vi "Read & Write Visa.vi"(8 "error in (no error)":errorcluster, 10 "Message":string, 11 "VISA Refnum in":refnum<visa-resource-name>) -> (0 "error out":errorcluster, 2 "read buffer":string, 3 "VISA Refnum out":refnum<visa-resource-name>)   [LabVIEW 2022 SP3]
uses:
  42f06f77-e9dd-42f2-8331-d96ccd674586.vi
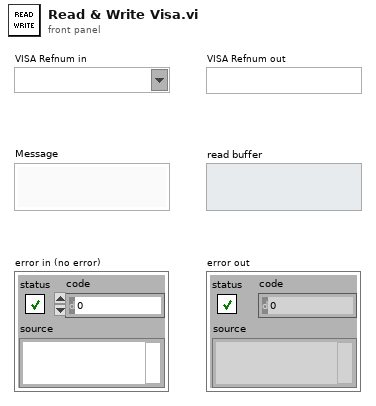
[diagram p1: front panel]
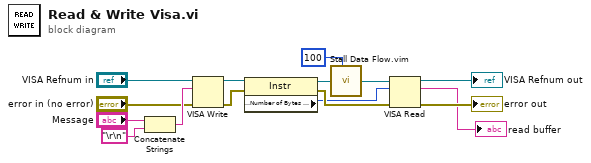
[diagram p0: block diagram]
diagram:
  n1 = Concatenate Strings("Message", "\r\n") -> (w4:string)
  n2 = VISA Write(VISA resource name="VISA Refnum in", write buffer=w4, error in (no error)="error in (no error)") -> (VISA resource name out=w6:refnum<visa-resource-name>, error out=w7:errorcluster)  [unwired: 1 out]
  n3 = property class="Instr"(reference=w6, error in=w7) -> (reference out=w8:refnum<visa-resource-name>, error out=w12:errorcluster, "Serial Settings:Number of Bytes at Serial Port"=w11:u32)
  n4 = call "Stall Data Flow.vim"("value in"=w8, "milliseconds to wait"=u32 100) -> ("value out"=w10:refnum<visa-resource-name>)  [unwired: 1 out]
  n5 = VISA Read(VISA resource name=w10, byte count=w11, error in (no error)=w12) -> (VISA resource name out=→"VISA Refnum out":refnum<visa-resource-name>, read buffer=→"read buffer":string, error out=→"error out":errorcluster)  [unwired: 1 out]
